vi "Time-Out.vi"(6 "External Clock":dbl, 7 "Time (S)":dbl) -> (3 "Timed Out":bool)   [LabVIEW 2020]
doc: "This is a timeout vi by Syed R. Use in a while loop to time out after a time set by the Time (S). A Tick Count timer must be added outside the loop to initialize. For usage, see the following: \nO:\\ENGE\\FTD\\Labview\\Source Code\\Shared VI's\\Time_Out_7.0\\Example of Time_out.vi"
panel:
  out "Clock In":dbl format="%#_8f"
  out "Clock Out":dbl format="%#_8f"
  # "INPUTS"
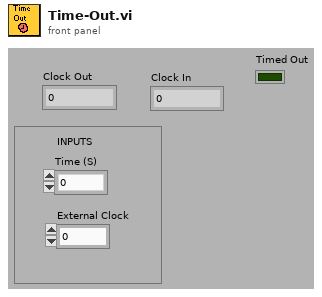
[diagram p1: front panel]
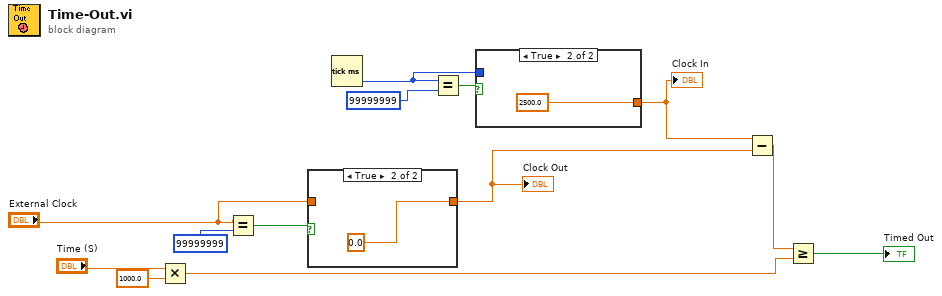
[diagram p0: block diagram]
diagram:
  n1 = Multiply(x="Time (S)", y=1000.0) -> (x*y=w2:dbl)
  n2 = Equal?(x="External Clock", y=u32 99999999) -> (x = y?=w11:bool)
  n3 = case shown="True" w11 {
    tunnel: "External Clock" -> [w14 _]
    tunnel: [w14 0.0 ("Numeric")] -> w7
    frame False {
    }
    frame True {
    }
  }
  "Clock Out" <- w7
  n4 = Tick Count (ms)() -> (millisecond timer value=w6:u32)
  n5 = Equal?(x=w6, y=u32 99999999) -> (x = y?=w9:bool)
  n6 = case shown="True" w9 {
    tunnel: [w16 2500.0 ("Numeric")] -> w5
    tunnel: w6 -> [w16 _]
    frame False {
    }
    frame True {
    }
  }
  "Clock In" <- w5
  n7 = Subtract(x=w5, y=w7) -> (x-y=w12:dbl)
  n8 = Greater Or Equal?(x=w12, y=w2) -> (x >= y?=→"Timed Out":bool)
